vi "DialogToDisplay.vi"(1 "Numeric":i32) -> (0 "Numeric 2":i32)   [LabVIEW 2011]
panel:
  out "?":string
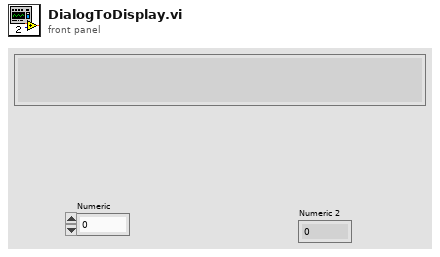
[diagram p1: front panel]
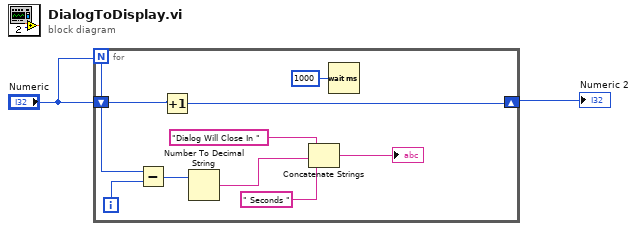
[diagram p0: block diagram]
diagram:
  n1 = for {
    N: "Numeric" -> [w7]
    shift-right: [w3] -> w1
    shift-left: "Numeric" -> [w4]
    i -> [w6]
    n2 = Subtract(x=w7, y=w6) -> (x-y=w5:i32)
    n3 = Increment(x=w4) -> (x+1=w3:i32)
    n4 = Number To Decimal String(number=w5) -> (decimal integer string=w10:string)  [unwired: 1 out]
    n5 = Concatenate Strings("Dialog Will Close In ", w10, " Seconds ") -> (→"?":string)
    n6 = Wait (ms)(milliseconds to wait=u32 1000) -> ()  [unwired: 1 out]
  }
  "Numeric 2" <- w1
